vi "Traceability_Code.vi"(7 "Return Data [ASR]":variant[][](array[variant]), 8 "error in (no error)":errorcluster, 9 "Return Data":variant[][](array[variant]), 10 "RFID":string, 11 "Ref in":T1={"MS SQL Connection"=refnum, "UDL File"=path "", "Time"="", "DCODE"="", "WIP+1"=0, "MC No?"=0, "POKAYOKE?"=FALSE, "Expected Result"="", "Result [Status]"="", "Clock"=0.0, "RFID"="", "WIP Queue"=refnum, "TS Parameter"={"ProfitCenterCode"="", "LineCode"="", "WorkOrderNumber"="", "Model"="", "Model_with_Prefix"="", "VendorCode"="", "SetParameterDateCode"="", "PokaYoke"=0, "Target"=1, "Live_DateCode"="", "CustomerPartNumber"="", "Hand"="", "sBarcode"=FALSE, "FCA"=0, "Ent_Stamp"=timestamp(0 s since 1904-01-01), "STS_CD"=0.0}, "Data_Queue"=[], "RFID Serial No."=""} {"TS Parameter"."FCA" format="%01d"; "TS Parameter"."Target" min=1 max=100000; "TS Parameter"."PokaYoke" min=0 max=1}) -> (0 "error out":errorcluster, 1 "TS_BSC":i32, 2 "TS_Message":string, 3 "Ref Out":T1={"MS SQL Connection"=refnum, "UDL File"=path "", "Time"="", "DCODE"="", "WIP+1"=0, "MC No?"=0, "POKAYOKE?"=FALSE, "Expected Result"="", "Result [Status]"="", "Clock"=0.0, "RFID"="", "WIP Queue"=refnum, "TS Parameter"={"ProfitCenterCode"="", "LineCode"="", "WorkOrderNumber"="", "Model"="", "Model_with_Prefix"="", "VendorCode"="", "SetParameterDateCode"="", "PokaYoke"=0, "Target"=1, "Live_DateCode"="", "CustomerPartNumber"="", "Hand"="", "sBarcode"=FALSE, "FCA"=0, "Ent_Stamp"=timestamp(0 s since 1904-01-01), "STS_CD"=0.0}, "Data_Queue"=[], "RFID Serial No."=""} {"TS Parameter"."FCA" format="%01d"; "TS Parameter"."Target" min=1 max=100000; "TS Parameter"."PokaYoke" min=0 max=1}, 4 "Message":picture, 5 "Act Count":i32)   [LabVIEW 2020]
uses:
  Controls/TD SQL.ctl
  <vilib>/addons/database/Connection.llb/Conn ObjectReference.ctl
  Controls/WIP_State.ctl
  Controls/TS_Parameter.ctl
  Controls/Msg_Type.ctl
  MS SQL/MS_Global.vi
  <vilib>/addons/database/NI_Database_API.lvlib
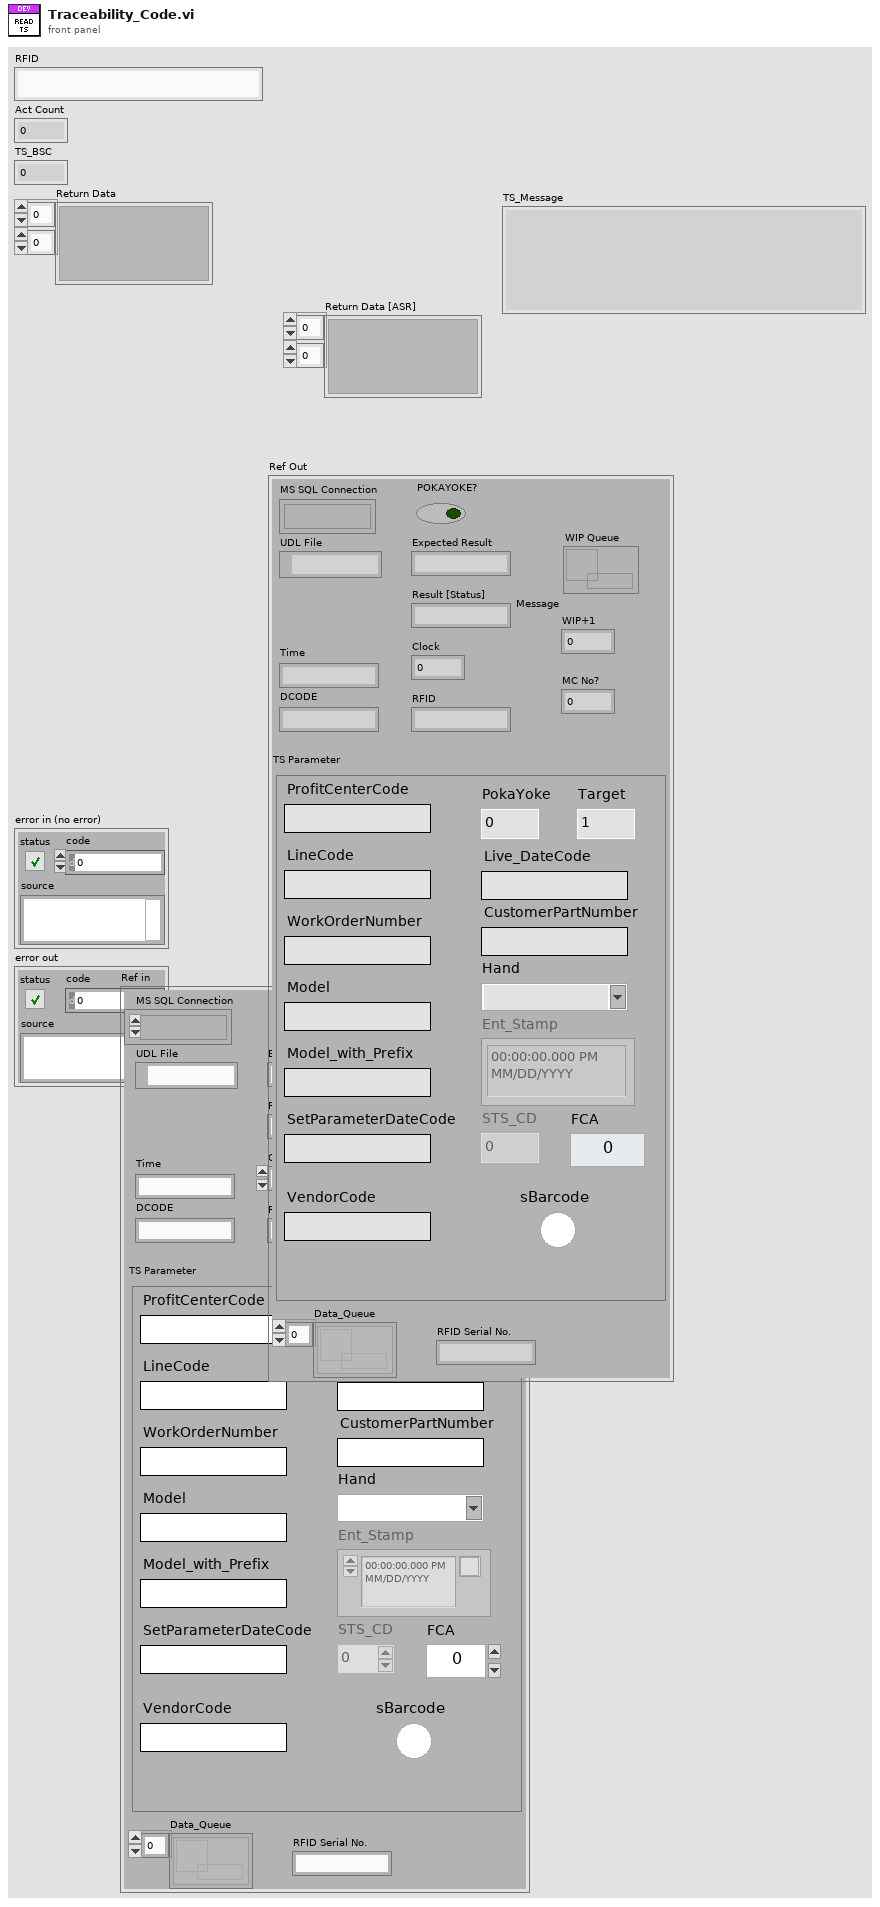
[diagram p1: front panel]
types:
  T1 = typedef "TD SQL.ctl" = cluster{"MS SQL Connection":T2, "UDL File":path, "Time":string, "DCODE":string, "WIP+1":i64, "MC No?":i32, "POKAYOKE?":bool, "Expected Result":string, "Result [Status]":string, "Clock":dbl, "RFID":string, "WIP Queue":refnum<queue>, "TS Parameter":T3, "Data_Queue":refnum<queue>[], "RFID Serial No.":string}
  T2 = typedef "NI_Database_API.lvlib/Conn ObjectReference.ctl" = refnum<k1>
  T3 = typedef "TS_Parameter.ctl" = cluster{"ProfitCenterCode":string, "LineCode":string, "WorkOrderNumber":string, "Model":string, "Model_with_Prefix":string, "VendorCode":string, "SetParameterDateCode":string, "PokaYoke":i32, "Target":i32, "Live_DateCode":string, "CustomerPartNumber":string, "Hand":string, "sBarcode":bool, "FCA":i32, "Ent_Stamp":timestamp, "STS_CD":dbl}
  T4 = cluster{"Text Color":u32, "Background Color":u32}
  T5 = typedef "WIP Limit.ctl" = cluster{"OP10":T6, "OP20A":T6, "OP20B":T6, "OP20C":T6, "OP20D":T6, "OP30":T6}
  T6 = typedef "WIP_old.ctl" = i64
  T7 = typedef "WIP_ref.ctl" = cluster{"WIP 1":refnum<vi>, "WIP 2":refnum<vi>, "WIP 3":refnum<vi>}
  T8 = typedef "LVTextColorsTypeDef.ctl" = cluster{"Text Color":u32, "Background Color":u32}
  T9 = typedef "Msg_Type.ctl" = enum16{"Normal", "Pass", "Fail", "Fault", "User", "Bypass", "Fail Save"}
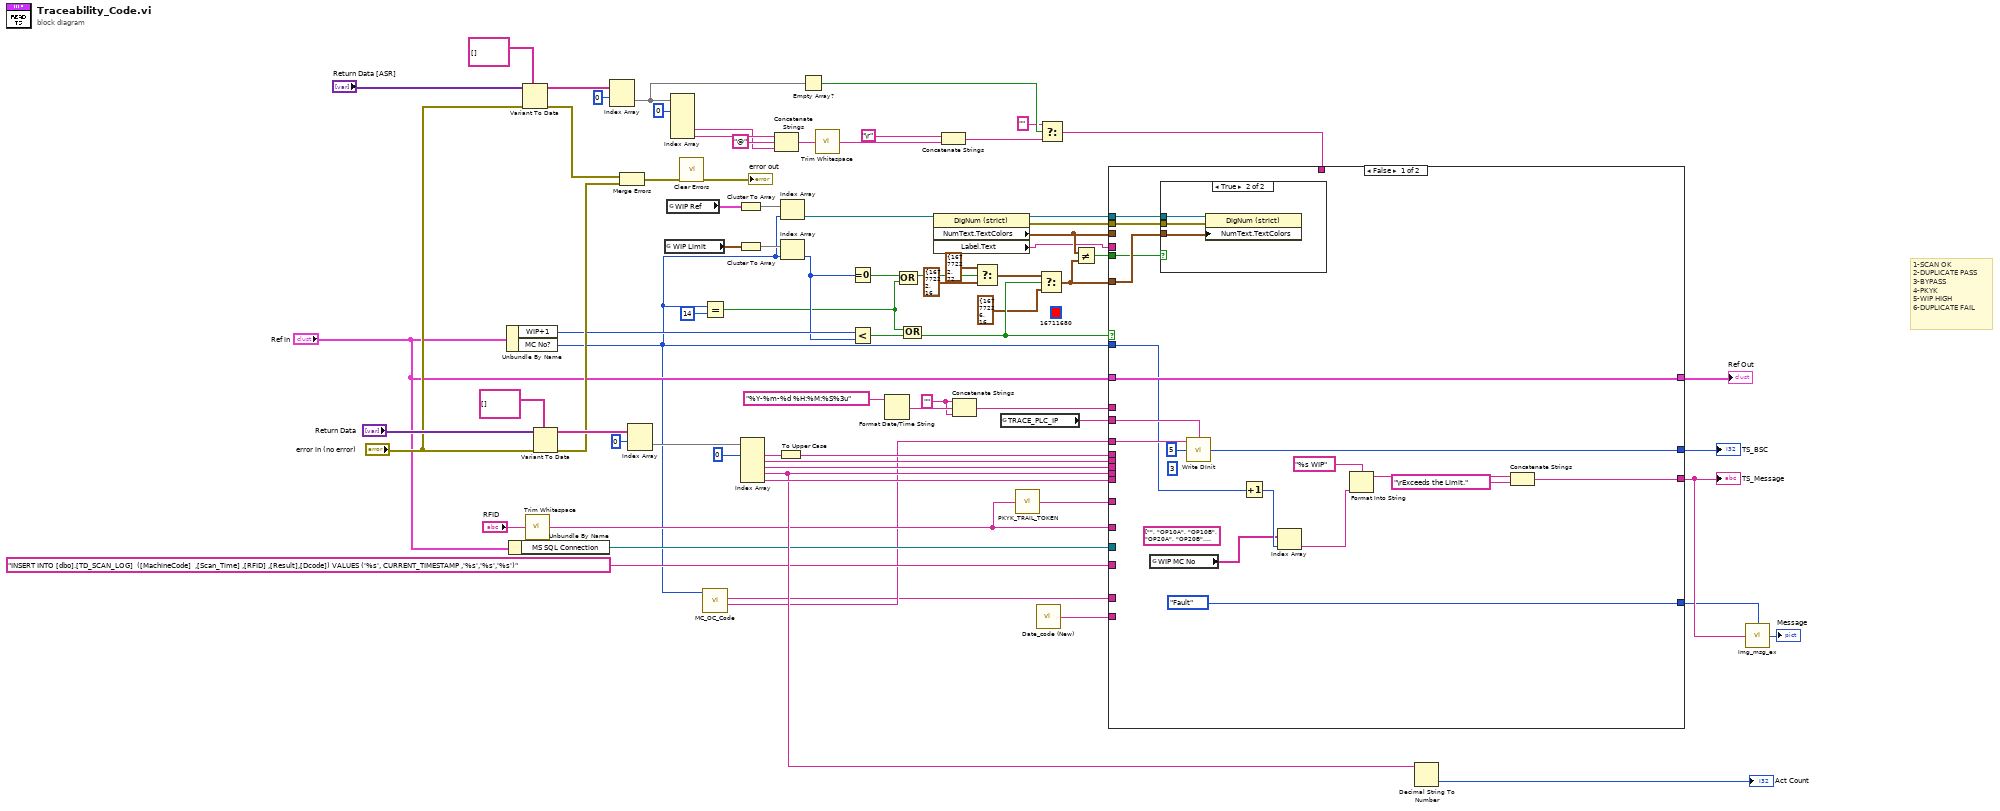
[diagram p0: block diagram]
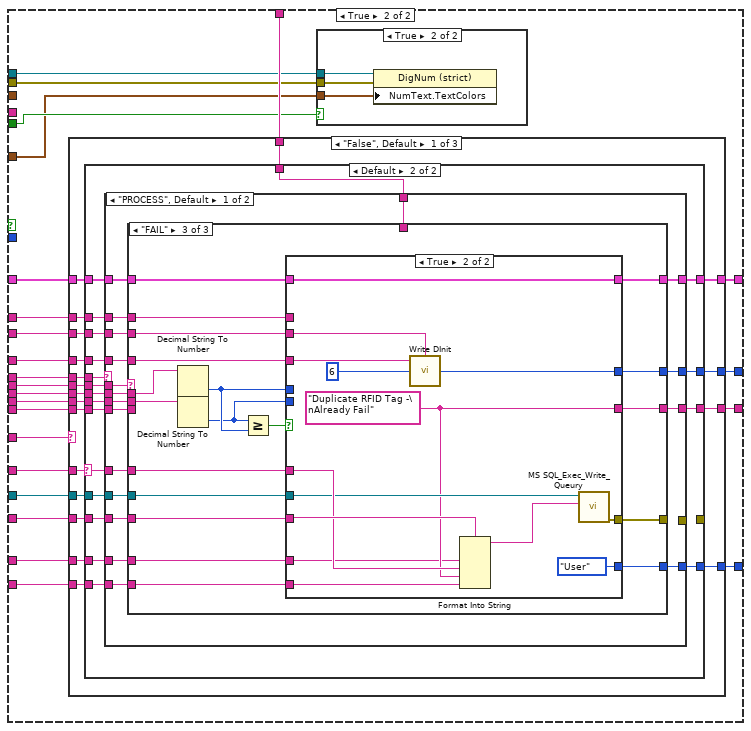
[diagram p3: hidden frame]
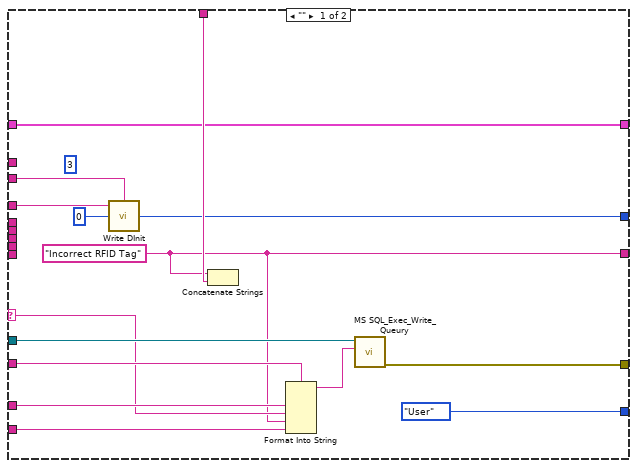
[diagram p5: hidden frame]
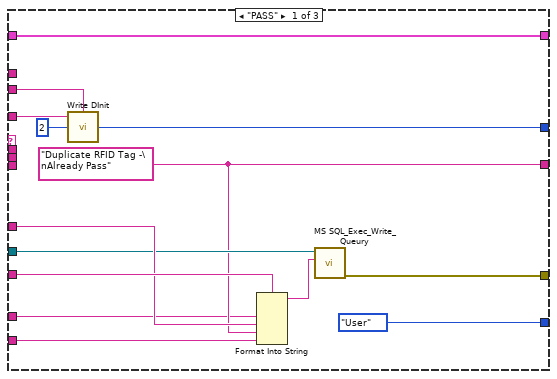
[diagram p6: hidden frame]
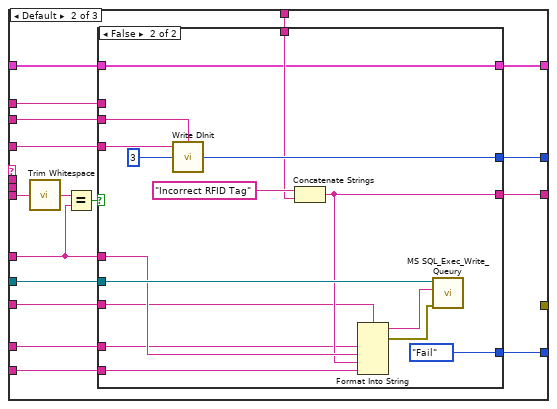
[diagram p7: hidden frame]
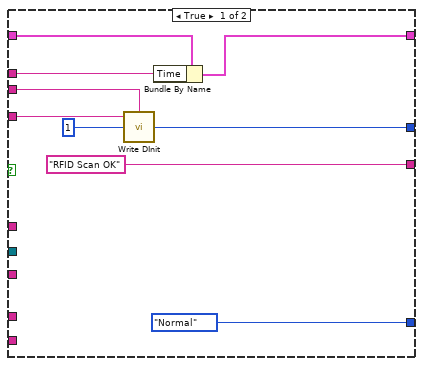
[diagram p8: hidden frame]
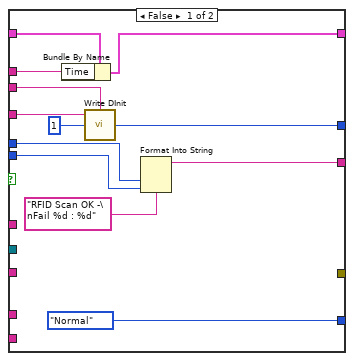
[diagram p9: hidden frame]
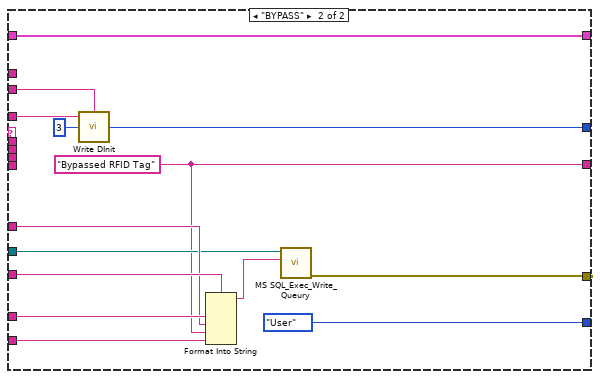
[diagram p10: hidden frame]
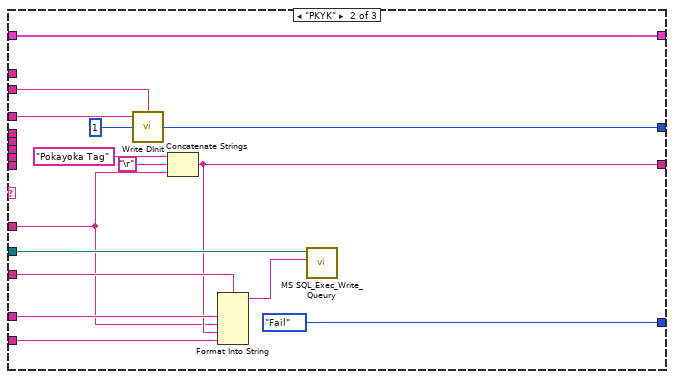
[diagram p11: hidden frame]
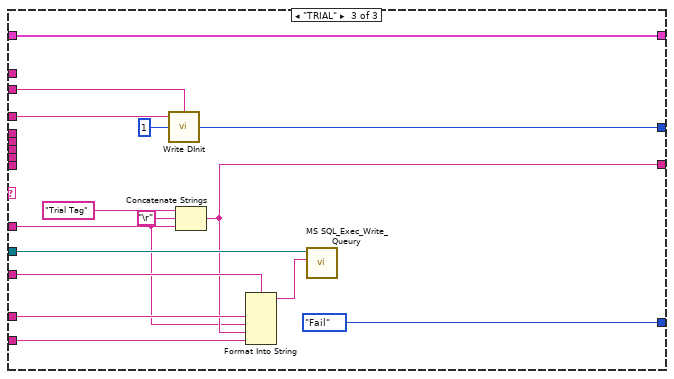
[diagram p12: hidden frame]
diagram:
  (unwired) u32 16711680 ("Selection Color")
  w35 = "" ("string")
  # "1-SCAN OK\n2-DUPLICATE PASS\n3-BYPASS\n4-PKYK\n5-WIP HIGH\n6-DUPLICATE FAIL"
  n1 = Unbundle By Name("Ref in") -> ("WIP+1"=w27:i64, "MC No?"=w4:i32)
  n2 = Unbundle By Name("Ref in") -> ("MS SQL Connection"=w62:T2)
  n3 = Variant To Data(error in="error in (no error)", type=string[][] [] ("Recent Data"), Variant="Return Data [ASR]") -> (data=w46:string[][], error out=w50:errorcluster)
  n4 = call <vilib>:"Trim Whitespace.vi"("string"="RFID") -> ("trimmed string"=w7:string)  [unwired: 1 in]
  n5 = Variant To Data(error in="error in (no error)", type=string[][] [] ("Recent Data"), Variant="Return Data") -> (data=w69:string[][], error out=w66:errorcluster)
  n6 = Index Array(array=w46, index (row)=0) -> (element=w45:string[])  [unwired: 1 in]
  n7 = Merge Errors(w50, w66) -> (w51:errorcluster)
  n8 = Index Array(array=w69, index (row)=0) -> (element=w34:string[])  [unwired: 1 in]
  n9 = global read "MS_Global.vi" "WIP Limit"() -> (w29:T5)
  n10 = global read "MS_Global.vi" "WIP Ref"() -> (w25:T7)
  n11 = Index Array(array=w45, index #1=0 ("index")) -> (element #4=w53:string, element #5=w55:string)  [unwired: 4 in, 3 out]
  n12 = call <vilib>:"Clear Errors.vi"("error in (no error)"=w51) -> ("error out"=→"error out":errorcluster)  [unwired: 5 in, 1 out]
  n13 = Equal?(x=w4, y=14) -> (x = y?=w11:bool)
  n14 = call "MC_OC_Code.vi"("index"=w4) -> ("TS CODE TAG"=w3:string, "Machine Code"=w2:string)  [unwired: 4 in, 5 out]
  n15 = Cluster To Array(cluster=w25) -> (array=w26:refnum<vi>[])
  n16 = Cluster To Array(cluster=w29) -> (array=w28:T6[])
  n17 = Index Array(array=w34, index #1=0 ("index")) -> (element #1=w64:string, element #2=w77:string, element #3=w71:string, element #4=w73:string, element #5=w76:string)  [unwired: 4 in]
  n18 = Concatenate Strings(w55, "@" ("string"), w53) -> (w52:string)
  n19 = To Upper Case(1:w64) -> (0:w63:string)
  n20 = Index Array(array=w26, index=w4) -> (element=w24:refnum<vi>)
  n21 = Index Array(array=w28, index=w4) -> (element=w21:T6)
  n22 = Empty Array?(array=w45) -> (empty?=w44:bool)
  n23 = call <vilib>:"Trim Whitespace.vi"("string"=w52) -> ("trimmed string"=w47:string)  [unwired: 1 in]
  n24 = Equal To 0?(x=w21) -> (x = 0?=w20:bool)
  n25 = Less?(x=w27, y=w21) -> (x < y?=w19:bool)
  n26 = Format Date/Time String(time format string (%c)="%Y-%m-%d %H:%M:%S%3u") -> (date/time string=w38:string)  [unwired: 2 in]
  n27 = Compound Arithmetic op=OR(w20, w11) -> (w13:bool)
  n28 = Compound Arithmetic op=OR(w11, w19) -> (w12:bool)
  n29 = property class="DigNum (strict)"(reference=w24) -> (reference out=w23:refnum<vi>, error out=w22:errorcluster, "NumText.TextColors"=w16:T8, "Label.Text"=w1:string)  [unwired: 1 in]
  n30 = Concatenate Strings("\r", w47) -> (w42:string)
  n31 = Concatenate Strings(w35, w38, w35) -> (w36:string)
  n32 = Select(t=T4 {"Text Color"=16777222, "Background Color"=7274306} ("Numeric Text.Text Colors"), s=w13, f=T4 {"Text Color"=16777222, "Background Color"=16777216} ("Numeric Text.Text Colors")) -> (s? t:f=w18:T4)
  n33 = global read "MS_Global.vi" "TRACE_PLC_IP"() -> (w5:string)
  n34 = call "PKYK_TRAIL_TOKEN.vi"("RFID In"=w7) -> ("PKYK?TRAIL"=w6:string)
  n35 = call "Date_code (New).vi"() -> ("Date Code"=w30:string)  [unwired: 14 in, 1 out]
  n36 = Select(t=w18, s=w12, f=T4 {"Text Color"=16777226, "Background Color"=16711680} ("Numeric Text.Text Colors")) -> (s? t:f=w17:T4)
  n37 = Select(t="", s=w44, f=w42) -> (s? t:f=w41:string)
  n38 = Not Equal?(x=w16, y=w17) -> (x != y?=w15:bool)
  n39 = case shown="False" w12 {
    tunnel: w77 -> [_ w121]
    tunnel: w76 -> [_ w120]
    tunnel: w73 -> [_ w119]
    tunnel: [w93 w118] -> w72
    tunnel: w71 -> [_ w117]
    tunnel: w63 -> [_ w116]
    tunnel: w62 -> [_ w115]
    tunnel: w2 -> [_ w114]
    tunnel: "INSERT INTO [dbo].[TD_SCAN_LOG]  ([MachineCode]  ,[Scan_Time] ,[RFID] ,[Result],[Dcode]) VALUES ('%s', CURRENT_TIMESTAMP ,'%s','%s','%s')" ("format string") -> [_ w113]
    tunnel: w3 -> [w92 w112]
    tunnel: w41 -> [_ w111]
    tunnel: "Ref in" -> [w94 w110]
    tunnel: [w94 w109] -> w37
    tunnel: w36 -> [_ w108]
    tunnel: [w89 w107] -> w33
    tunnel: [Msg_Type."Fault" ("Msg Type") w106] -> w32
    tunnel: w30 -> [_ w105]
    tunnel: w7 -> [_ w104]
    tunnel: w6 -> [_ w103]
    tunnel: w4 -> [w81 _]
    tunnel: w23 -> [w86 w102]
    tunnel: w16 -> [_ _]
    tunnel: w22 -> [w85 w101]
    tunnel: w17 -> [w84 w99]
    tunnel: w15 -> [w83 w100]
    tunnel: w5 -> [w82 w98]
    tunnel: w1 -> [_ _]
    frame False {
      (unwired) string[] ["", "OP10A", "OP10B", "OP20A", "OP20B", "OP30A", "OP30B", "OP30C", "OP40A", "OP40B", "OP50A", "OP50B", "OP60", "OP70", "OP80"] ("TS_CODE_TAG")
      (unwired) 3 ("TS_BSC")
      w93 = 5 ("TS_BSC")
      n40 = global read "MS_Global.vi" "WIP MC No"() -> (w78:string[])
      n41 = case shown="True" w83 {
        tunnel: w86 -> [_ w97]
        tunnel: w85 -> [_ w96]
        tunnel: w84 -> [_ w95]
        frame False {
        }
        frame True {
          n42 = property class="DigNum (strict)"(reference=w97, error in=w96, "NumText.TextColors"=w95) -> ()  [unwired: 2 out]
        }
      }
      n43 = call "Write DInit.vi"("Network Path"=w82, "Int"=w93, "Tag Name"=w92) -> ()  [unwired: 2 in]
      n44 = Increment(x=w81) -> (x+1=w79:i32)
      n45 = Index Array(array=w78, index=w79) -> (element=w80:string)
      n46 = Format Into String(format string="%s WIP" ("string"), w80) -> (resulting string=w87:string)  [unwired: 2 in, 1 out]
      n47 = Concatenate Strings(w87, "\rExceeds the Limit." ("string")) -> (w89:string)
    }
    frame True {
      n48 = case shown="\"False\", Default" w103 {
        tunnel: w121 -> [w143 _ _]
        tunnel: w120 -> [w142 _ _]
        tunnel: w119 -> [w141 _ _]
        tunnel: [w140 w308 w322] -> w118
        tunnel: w117 -> [w139 _ _]
        tunnel: w116 -> [w138 _ _]
        tunnel: w115 -> [w137 w317 w331]
        tunnel: w114 -> [w136 w316 w330]
        tunnel: w113 -> [w135 w315 w329]
        tunnel: w112 -> [w134 w307 w321]
        tunnel: w111 -> [w133 _ _]
        tunnel: w110 -> [w132 w314 w328]
        tunnel: [w131 w314 w328] -> w109
        tunnel: w108 -> [w130 _ _]
        tunnel: [w129 w313 w327] -> w107
        tunnel: [w128 Msg_Type."Fail" ("Msg Type") Msg_Type."Fail" ("Msg Type")] -> w106
        tunnel: w105 -> [w127 w311 w325]
        tunnel: w104 -> [w126 w306 w320]
        tunnel: w98 -> [w125 w304 w318]
        frame "False", Default {
          n49 = case shown="Default" w126 {
            selector: w126 -> [w148 w159]
            tunnel: w143 -> [_ w176]
            tunnel: w142 -> [_ w175]
            tunnel: w141 -> [_ w174]
            tunnel: [w144 w173] -> w129
            tunnel: [w145 w172] -> w140
            tunnel: w139 -> [_ w171]
            tunnel: w138 -> [_ w170]
            tunnel: w137 -> [w157 w169]
            tunnel: [w156 _] -> _
            tunnel: w136 -> [w155 w167]
            tunnel: w135 -> [w154 w168]
            tunnel: w134 -> [w146 w166]
            tunnel: w133 -> [w152 w165]
            tunnel: w132 -> [w151 w164]
            tunnel: w130 -> [_ w163]
            tunnel: [w151 w162] -> w131
            tunnel: [Msg_Type."User" ("Msg Type") w161] -> w128
            tunnel: w127 -> [w149 w160]
            tunnel: w125 -> [w147 w158]
            frame "" {
              (unwired) 3 ("TS_BSC")
              w145 = 0 ("TS_BSC")
              w144 = "Incorrect RFID Tag"
              n50 = call "Write DInit.vi"("Network Path"=w147, "Int"=w145, "Tag Name"=w146) -> ()  [unwired: 2 in]
              n51 = Concatenate Strings(w144, w152) -> ()  [unwired: 1 out]
              n52 = Format Into String(format string=w154, w155, w148, w144, w149) -> (resulting string=w153:string)  [unwired: 2 in, 1 out]
              n53 = call "MS SQL_Exec_Write_Queury.vi"("Query"=w153, "Refnum in"=w157) -> ("error out"=w156:errorcluster)  [unwired: 8 in, 1 out]
            }
            frame Default {
              n54 = case shown="\"PROCESS\", Default" w170 {
                tunnel: w176 -> [w194 _]
                tunnel: w175 -> [w193 _]
                tunnel: w159 -> [w192 w300]
                tunnel: w174 -> [w191 _]
                tunnel: [w190 w295] -> w173
                tunnel: [w189 w297] -> w172
                tunnel: w171 -> [w188 _]
                tunnel: w169 -> [w187 w299]
                tunnel: w168 -> [w186 w302]
                tunnel: w167 -> [w177 w301]
                tunnel: [_ w298] -> _
                tunnel: w166 -> [w185 w296]
                tunnel: w165 -> [w184 _]
                tunnel: w164 -> [w183 w294]
                tunnel: w163 -> [w182 _]
                tunnel: [w181 w294] -> w162
                tunnel: [w180 Msg_Type."User" ("Msg Type")] -> w161
                tunnel: w160 -> [w179 w292]
                tunnel: w158 -> [w178 w291]
                frame "PROCESS", Default {
                  n55 = case shown="\"FAIL\"" w194 {
                    tunnel: w188 -> [_ _ w264]
                    tunnel: w191 -> [_ _ w263]
                    tunnel: [w202 w224 w266] -> w189
                    tunnel: [w200 w223 w265] -> w190
                    tunnel: w192 -> [w205 w217 w258]
                    tunnel: w193 -> [_ w222 _]
                    tunnel: w187 -> [w204 w219 w261]
                    tunnel: [w203 _ w260] -> _
                    tunnel: w186 -> [w206 w218 w259]
                    tunnel: w185 -> [w201 w216 w257]
                    tunnel: w184 -> [_ w215 _]
                    tunnel: w183 -> [w199 w214 w256]
                    tunnel: w182 -> [_ w213 w255]
                    tunnel: [w199 w212 w254] -> w181
                    tunnel: [Msg_Type."User" ("Msg Type") w211 w253] -> w180
                    tunnel: w179 -> [w197 w210 w252]
                    tunnel: w178 -> [w196 w209 w249]
                    tunnel: w177 -> [w195 w208 w248]
                    frame "PASS" {
                      w200 = "Duplicate RFID Tag -\nAlready Pass"
                      w202 = 2 ("TS_BSC")
                      n56 = call "Write DInit.vi"("Network Path"=w196, "Int"=w202, "Tag Name"=w201) -> ()  [unwired: 2 in]
                      n57 = Format Into String(format string=w206, w195, w205, w200, w197) -> (resulting string=w207:string)  [unwired: 2 in, 1 out]
                      n58 = call "MS SQL_Exec_Write_Queury.vi"("Query"=w207, "Refnum in"=w204) -> ("error out"=w203:errorcluster)  [unwired: 8 in, 1 out]
                    }
                    frame Default {
                      n59 = call <vilib>:"Trim Whitespace.vi"("string"=w222) -> ("trimmed string"=w221:string)  [unwired: 1 in]
                      n60 = Equal?(x=w221, y=w217) -> (x = y?=w220:bool)
                      n61 = case shown="False" w220 {
                        tunnel: [w231 w243] -> w224
                        tunnel: ["RFID Scan OK" w240] -> w223
                        tunnel: w219 -> [_ w246]
                        tunnel: w218 -> [_ w235]
                        tunnel: w217 -> [_ w245]
                        tunnel: w216 -> [w232 w242]
                        tunnel: w215 -> [_ w241]
                        tunnel: w214 -> [w229 w239]
                        tunnel: w213 -> [w228 _]
                        tunnel: [w227 w239] -> w212
                        tunnel: [Msg_Type."Normal" ("Msg Type") Msg_Type."Fail" ("Msg Type")] -> w211
                        tunnel: w210 -> [_ w237]
                        tunnel: w209 -> [w225 w234]
                        tunnel: w208 -> [_ w233]
                        frame True {
                          w231 = 1 ("TS_BSC")
                          n62 = call "Write DInit.vi"("Network Path"=w225, "Int"=w231, "Tag Name"=w232) -> ()  [unwired: 2 in]
                          n63 = Bundle By Name(cluster=w229, "Time"=w228) -> (w227:T1)
                        }
                        frame False {
                          w243 = 3 ("TS_BSC")
                          n64 = call "Write DInit.vi"("Network Path"=w234, "Int"=w243, "Tag Name"=w242) -> ()  [unwired: 2 in]
                          n65 = Concatenate Strings("Incorrect RFID Tag", w241) -> (w240:string)
                          n66 = Format Into String(format string=w235, w233, w245, w240, w237) -> (resulting string=w247:string, error out=w236:errorcluster)  [unwired: 2 in]
                          n67 = call "MS SQL_Exec_Write_Queury.vi"("error in (no error)"=w236, "Query"=w247, "Refnum in"=w246) -> ()  [unwired: 7 in, 2 out]
                        }
                      }
                    }
                    frame "FAIL" {
                      n68 = Decimal String To Number(string=w264) -> (number=w251:i32)  [unwired: 2 in, 1 out]
                      n69 = Decimal String To Number(string=w263) -> (number=w250:i32)  [unwired: 2 in, 1 out]
                      n70 = Greater Or Equal?(x=w250, y=w251) -> (x >= y?=w262:bool)
                      n71 = case shown="True" w262 {
                        tunnel: [w276 w285] -> w266
                        tunnel: [w268 w283] -> w265
                        tunnel: w261 -> [_ w287]
                        tunnel: [_ w286] -> w260
                        tunnel: w259 -> [_ w289]
                        tunnel: w258 -> [_ w288]
                        tunnel: w257 -> [w277 w284]
                        tunnel: w256 -> [w275 w282]
                        tunnel: w255 -> [w274 _]
                        tunnel: [w273 w282] -> w254
                        tunnel: [Msg_Type."Normal" ("Msg Type") Msg_Type."User" ("Msg Type")] -> w253
                        tunnel: w252 -> [_ w280]
                        tunnel: w251 -> [w270 _]
                        tunnel: w250 -> [w269 _]
                        tunnel: w249 -> [w267 w279]
                        tunnel: w248 -> [_ w278]
                        frame False {
                          w276 = 1 ("TS_BSC")
                          n72 = Bundle By Name(cluster=w275, "Time"=w274) -> (w273:T1)
                          n73 = call "Write DInit.vi"("Network Path"=w267, "Int"=w276, "Tag Name"=w277) -> ()  [unwired: 2 in]
                          n74 = Format Into String(format string="RFID Scan OK -\nFail %d : %d", w270, w269) -> (resulting string=w268:string)  [unwired: 2 in, 1 out]
                        }
                        frame True {
                          w283 = "Duplicate RFID Tag -\nAlready Fail"
                          w285 = 6 ("TS_BSC")
                          n75 = call "Write DInit.vi"("Network Path"=w279, "Int"=w285, "Tag Name"=w284) -> ()  [unwired: 2 in]
                          n76 = Format Into String(format string=w289, w278, w288, w283, w280) -> (resulting string=w290:string)  [unwired: 2 in, 1 out]
                          n77 = call "MS SQL_Exec_Write_Queury.vi"("Query"=w290, "Refnum in"=w287) -> ("error out"=w286:errorcluster)  [unwired: 8 in, 1 out]
                        }
                      }
                    }
                  }
                }
                frame "BYPASS" {
                  w297 = 3 ("TS_BSC")
                  w295 = "Bypassed RFID Tag"
                  n78 = call "Write DInit.vi"("Network Path"=w291, "Int"=w297, "Tag Name"=w296) -> ()  [unwired: 2 in]
                  n79 = Format Into String(format string=w302, w301, w300, w295, w292) -> (resulting string=w303:string)  [unwired: 2 in, 1 out]
                  n80 = call "MS SQL_Exec_Write_Queury.vi"("Query"=w303, "Refnum in"=w299) -> ("error out"=w298:errorcluster)  [unwired: 8 in, 1 out]
                }
              }
            }
          }
        }
        frame "PKYK" {
          w308 = 1 ("TS_BSC")
          n81 = call "Write DInit.vi"("Network Path"=w304, "Int"=w308, "Tag Name"=w307) -> ()  [unwired: 2 in]
          n82 = Concatenate Strings("Pokayoka Tag", "\r", w306) -> (w313:string)
          n83 = Format Into String(format string=w315, w316, w306, w313, w311) -> (resulting string=w309:string)  [unwired: 2 in, 1 out]
          n84 = call "MS SQL_Exec_Write_Queury.vi"("Query"=w309, "Refnum in"=w317) -> ()  [unwired: 8 in, 2 out]
        }
        frame "TRIAL" {
          w322 = 1 ("TS_BSC")
          n85 = call "Write DInit.vi"("Network Path"=w318, "Int"=w322, "Tag Name"=w321) -> ()  [unwired: 2 in]
          n86 = Concatenate Strings("Trial Tag", "\r", w320) -> (w327:string)
          n87 = Format Into String(format string=w329, w330, w320, w327, w325) -> (resulting string=w323:string)  [unwired: 2 in, 1 out]
          n88 = call "MS SQL_Exec_Write_Queury.vi"("Query"=w323, "Refnum in"=w331) -> ()  [unwired: 8 in, 2 out]
        }
      }
      n89 = case shown="True" w100 {
        tunnel: w102 -> [_ w124]
        tunnel: w101 -> [_ w123]
        tunnel: w99 -> [_ w122]
        frame False {
        }
        frame True {
          n90 = property class="DigNum (strict)"(reference=w124, error in=w123, "NumText.TextColors"=w122) -> ()  [unwired: 2 out]
        }
      }
    }
  }
  "TS_BSC" <- w72
  "TS_Message" <- w33
  "Ref Out" <- w37
  n91 = Decimal String To Number(string=w73) -> (number=→"Act Count":i32)  [unwired: 2 in, 1 out]
  n92 = call "Img_msg_ex.vi"("Msg Type"=w32, "Message In"=w33) -> ("Message"=→"Message":picture)  [unwired: 2 in]
